vi "results2candyIndicators.vi"(7 "conf":sgl, 8 "error in (no error)":errorcluster, 10 "results":T3[](array[typedef]), 11 "img in":T2) -> (0 "error out":errorcluster, 2 "ui array":T1(array[cluster]), 3 "img out":T2)   [LabVIEW 2024]
uses:
  toolkit/rectangularDetectedObject.ctl
  toolkit/transformCv.lvclass
  <vilib>/vision/Image Controls.llb/IMAQ Image.ctl
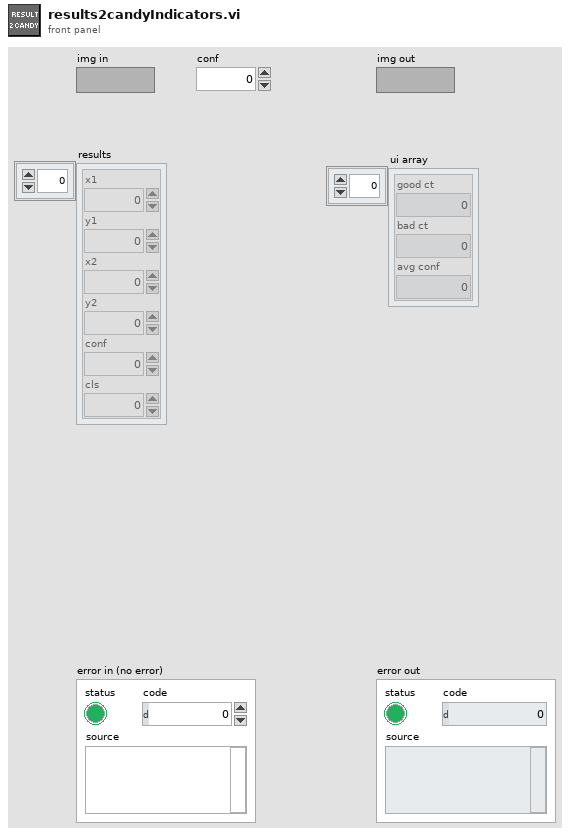
[diagram p1: front panel]
types:
  T1 = cluster{"good ct":i32, "bad ct":i32, "avg conf":dbl}[]
  T2 = typedef "IMAQ Image.ctl" = refnum<image>
  T3 = typedef "transformCv.lvclass/rectangularDetectedObject.ctl" = cluster{"x1":sgl, "y1":sgl, "x2":sgl, "y2":sgl, "conf":sgl, "cls":i32}
  T4 = cluster{"Desired Font (Application)":enum16{"User-specified Font", "Application Font", "System Font", "Dialog Font"}, "[User-specified Font]":cluster{"Font Name":string, "Size":i16, "Strikeout?":bool, "Italic?":bool, "Underline?":bool, "Outline?":bool, "Shadow?":bool, "Bold?":bool, "Rotation Angle":dbl}, "Horizontal Alignment":i16, "Vertical Alignment":i16}
  T5 = cluster{"Left":i32, "Top":i32, "Right":i32, "Bottom":i32}
  T6 = cluster{"good ct":i32, "bad ct":i32, "avg conf":dbl}
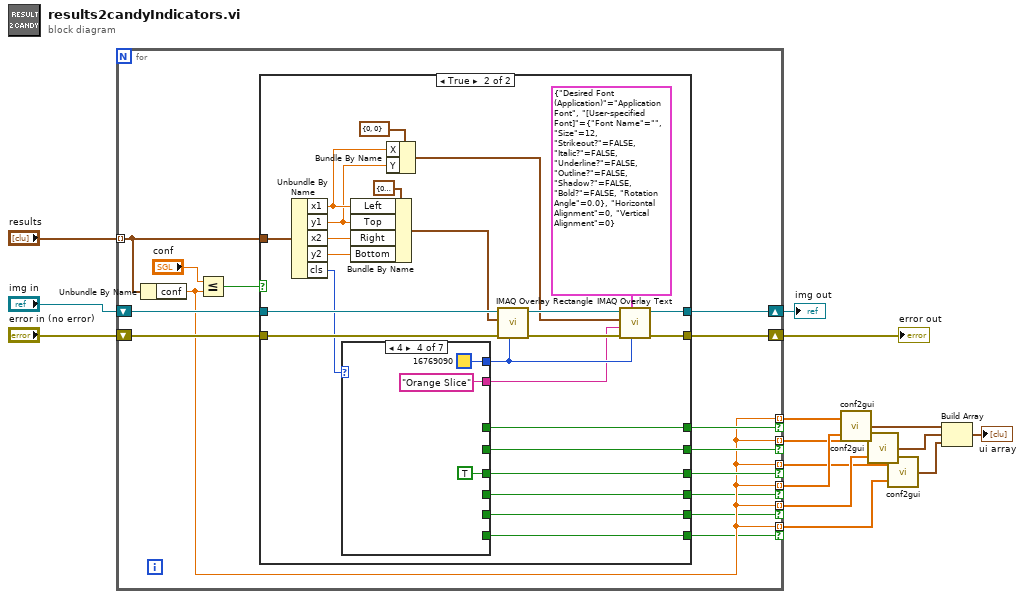
[diagram p0: block diagram]
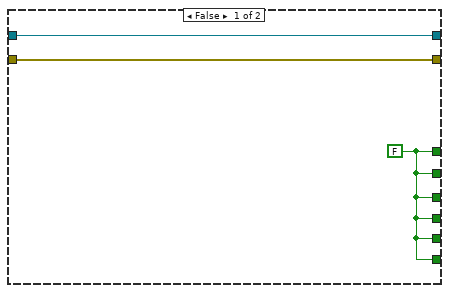
[diagram p2: hidden frame]
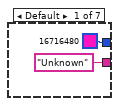
[diagram p3: hidden frame]
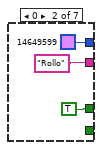
[diagram p4: hidden frame]
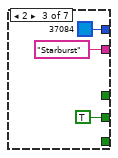
[diagram p5: hidden frame]
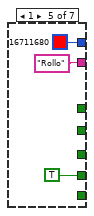
[diagram p6: hidden frame]
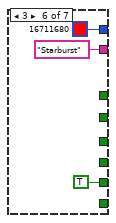
[diagram p7: hidden frame]
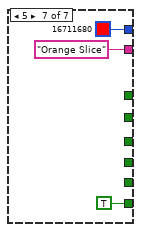
[diagram p8: hidden frame]
diagram:
  n1 = for {
    shift-right: [w27] -> w12
    shift-left: "img in" -> [w29]
    shift-right: [w26] -> w11
    shift-left: "error in (no error)" -> [w28]
    tunnel: "results" -> [w24] mode=indexing
    tunnel: [w19] -> w6 mode=indexing if=w22
    tunnel: [w19] -> w10 mode=indexing if=w21
    tunnel: [w19] -> w8 mode=indexing if=w20
    tunnel: [w19] -> w9 mode=indexing if=w18
    tunnel: [w19] -> w7 mode=indexing if=w17
    tunnel: [w19] -> w5 mode=indexing if=w16
    n2 = Unbundle By Name(w24) -> ("conf"=w19:sgl)
    n3 = Less Or Equal?(x="conf", y=w19) -> (x <= y?=w25:bool)
    n4 = case shown="True" w25 {
      tunnel: w29 -> [w32 w57]
      tunnel: w28 -> [w31 w56]
      tunnel: [w32 w47] -> w27
      tunnel: [w31 w46] -> w26
      tunnel: w24 -> [_ w53]
      tunnel: [w30 w38] -> w22
      tunnel: [w30 w37] -> w21
      tunnel: [w30 w36] -> w20
      tunnel: [w30 w35] -> w18
      tunnel: [w30 w34] -> w17
      tunnel: [w30 w33] -> w16
      frame False {
        w30 = FALSE ("defect")
      }
      frame True {
        n5 = Unbundle By Name(w53) -> ("x1"=w44:sgl, "y1"=w43:sgl, "x2"=w52:sgl, "y2"=w51:sgl, "cls"=w50:i32)
        n6 = case shown="4" w50 {
          tunnel: [u32 16716480 ("Color") u32 14649599 ("Color") u32 37084 ("Color") u32 16769090 ("Color") u32 16711680 ("Color") u32 16711680 ("Color") u32 16711680 ("Color")] -> w40
          tunnel: ["Unknown" ("String") "Rollo" ("String") "Starburst" ("String") "Orange Slice" ("String") "Rollo" ("String") "Starburst" ("String") "Orange Slice" ("String")] -> w39
          tunnel: [_ _ _ _ TRUE ("defect") _ _] -> w35
          tunnel: [_ _ _ TRUE ("defect") _ _ _] -> w38
          tunnel: [_ TRUE ("defect") _ _ _ _ _] -> w37
          tunnel: [_ _ TRUE ("defect") _ _ _ _] -> w36
          tunnel: [_ _ _ _ _ TRUE ("defect") _] -> w34
          tunnel: [_ _ _ _ _ _ TRUE ("defect")] -> w33
          frame Default {
          }
          frame 0 {
          }
          frame 2 {
          }
          frame 4 {
          }
          frame 1 {
          }
          frame 3 {
          }
          frame 5 {
          }
        }
        n7 = Bundle By Name(cluster=T5 {"Left"=0, "Top"=0, "Right"=0, "Bottom"=0} ("Rectangle"), "Left"=w44, "Top"=w43, "Right"=w52, "Bottom"=w51) -> (w54:T5)
        n8 = Bundle By Name(cluster=cluster{"X":i32, "Y":i32} {"X"=0, "Y"=0} ("Origin"), "X"=w44, "Y"=w43) -> (w42:cluster{"X":i32, "Y":i32})
        n9 = call "IMAQ Overlay Rectangle"("Color"=w40, "error in (no error)"=w56, "Rectangle"=w54, "Image"=w57) -> ("error out"=w48:errorcluster, "Image Out"=w49:T2)  [unwired: 6 in]
        n10 = call "IMAQ Overlay Text"("Text Color (black)"=w40, "Font, Size & Style"=T4 {"Desired Font (Application)"=enum."Application Font", "[User-specified Font]"={"Font Name"="", "Size"=12, "Strikeout?"=FALSE, "Italic?"=FALSE, "Underline?"=FALSE, "Outline?"=FALSE, "Shadow?"=FALSE, "Bold?"=FALSE, "Rotation Angle"=0.0}, "Horizontal Alignment"=0, "Vertical Alignment"=0}, "error in (no error)"=w48, "String"=w39, "Origin"=w42, "Image"=w49) -> ("error out"=w46:errorcluster, "Image Out"=w47:T2)  [unwired: 4 in]
      }
    }
  }
  "img out" <- w12
  "error out" <- w11
  n11 = call "conf2gui.vi"("bad conf"=w9, "good conf"=w10) -> ("ui info"=w4:T6)
  n12 = call "conf2gui.vi"("bad conf"=w7, "good conf"=w8) -> ("ui info"=w3:T6)
  n13 = call "conf2gui.vi"("bad conf"=w5, "good conf"=w6) -> ("ui info"=w2:T6)
  n14 = Build Array(w4, w3, w2) -> (→"ui array":T1)
